vi "Write Requested.vi"(8 "error in":errorcluster, 10 "Requested":bool, 11 "Output Timer in":refnum<class "Output Timer.lvclass">) -> (0 "error out":errorcluster, 3 "Output Timer out":refnum<class "Output Timer.lvclass">)   [LabVIEW 2013, in "Output Timer.lvclass"]
uses:
  Output Timer.lvclass
  Output Timer.lvclass/Output Timer.ctl
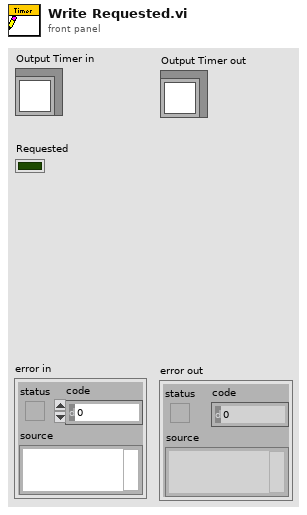
[diagram p1: front panel]
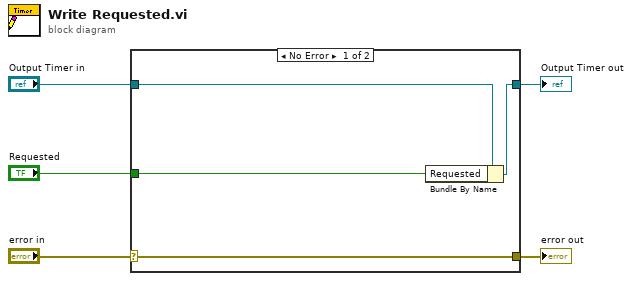
[diagram p0: block diagram]
diagram:
  n1 = case shown="No Error" "error in" {
    selector: "error in" -> [w9 w10]
    tunnel: [w9 w10] -> w4
    tunnel: [w7 w11] -> w2
    tunnel: "Output Timer in" -> [w8 w11]
    tunnel: "Requested" -> [w6 _]
    frame No Error {
      n2 = Bundle By Name(cluster=w8, "Requested"=w6) -> (w7:refnum<class "Output Timer.lvclass">)
    }
    frame Error {
    }
  }
  "error out" <- w4
  "Output Timer out" <- w2
